vi "Global Lens Driver.vi"() -> ()   [LabVIEW 2015]
panel:
  out "OK":bool
  in  "Current DC B":dbl
  in  "Current DC A":dbl
  in  "End VI":bool
  in  "Reset":bool
  in  "Run":bool
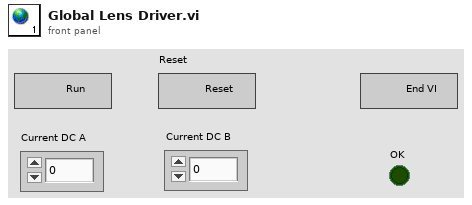
[diagram p1: front panel]
diagram:
